vi "plot_usr_seq.vi"(1 "User-defined sequence":string[][](table)) -> (0 "Sequence Preview":cluster{dbl[], dbl[]}[](graph))   [LabVIEW 2014]
panel:
  in  "Boolean":bool=TRUE
  out "Total sequence time (sec)":dbl
  out "vapor flow":dbl
  out "gas flow":dbl
  out "Pressure":dbl
  out "light up\ncurrent step":bool[](array[boolean])
  in  "Run sequence":bool
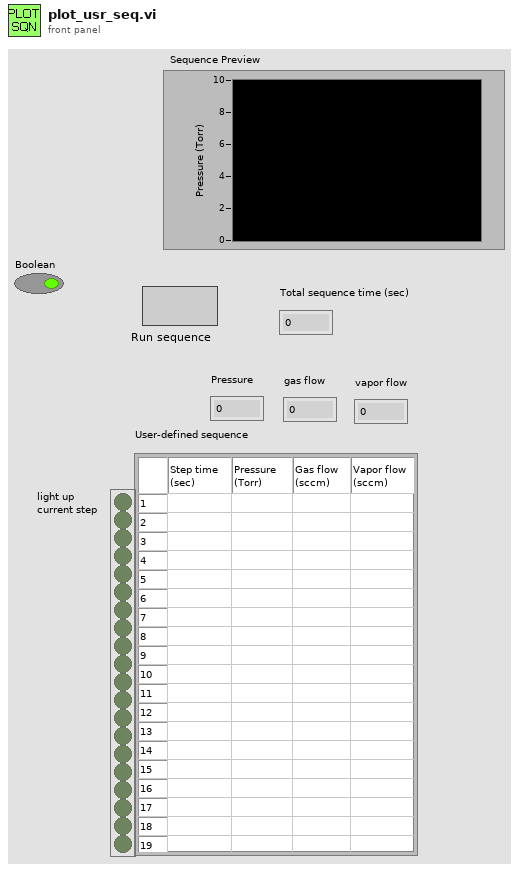
[diagram p1: front panel]
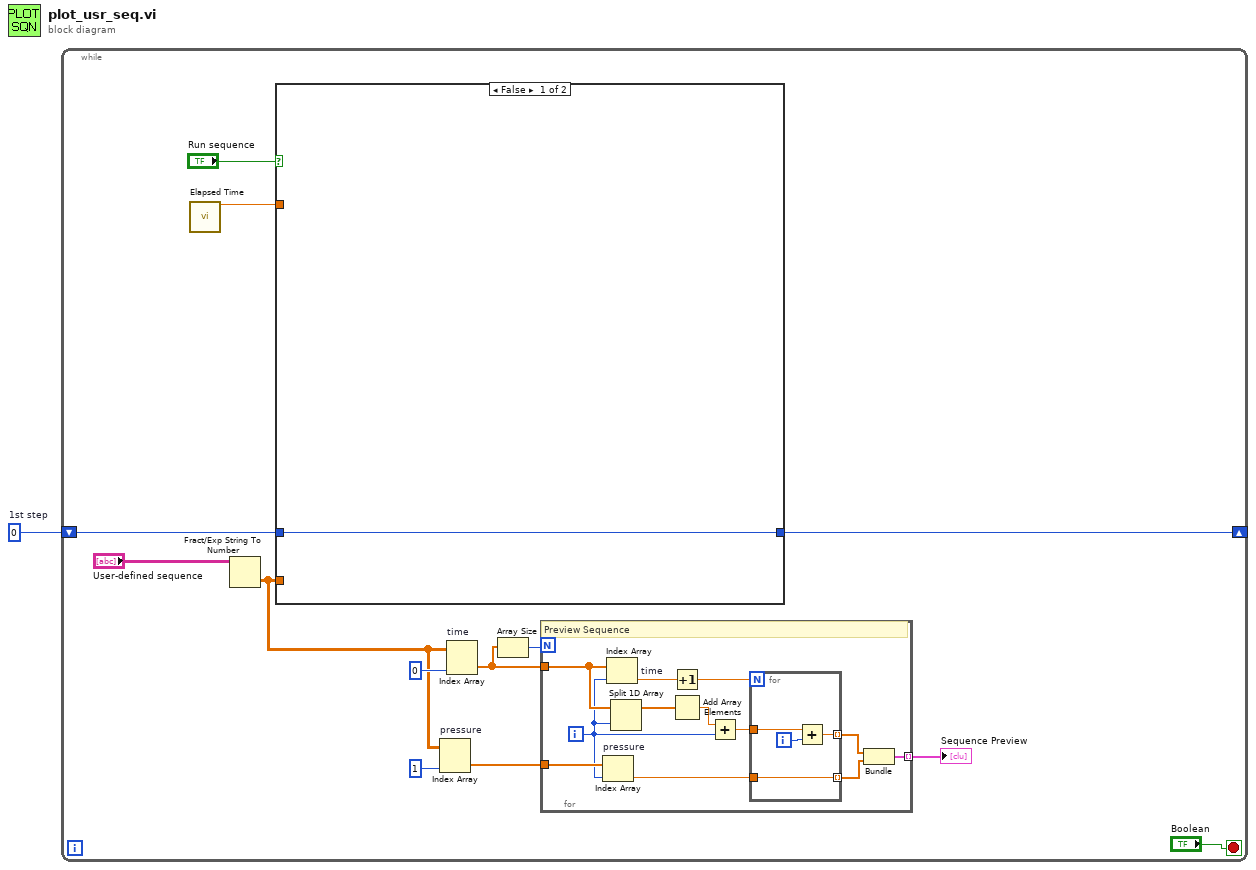
[diagram p0: block diagram]
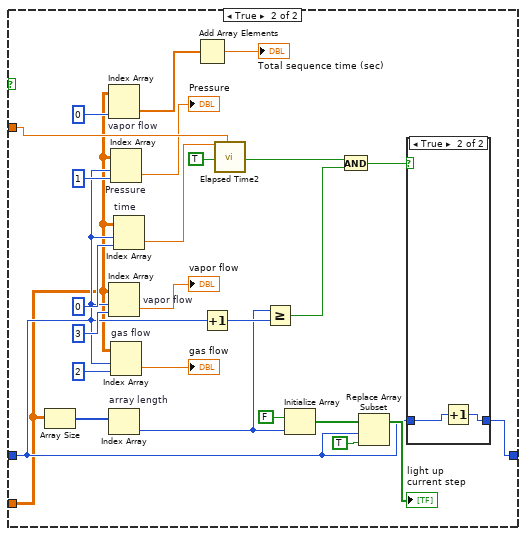
[diagram p2: hidden frame]
diagram:
  w1 = 0  # 1st step
  n1 = while {
    shift-right: [w13] -> _
    shift-left: w1 -> [w12]
    stop <- "Boolean" stop-if-true
    n2 = call "Elapsed Time"() -> ("Present (s)"=w14:dbl)  [unwired: 12 in, 7 out]
    n3 = Fract/Exp String To Number(string="User-defined sequence") -> (number=w6:dbl[][])  [unwired: 3 in, 1 out]
    n4 = case shown="False" "Run sequence" {
      tunnel: w14 -> [_ w35]
      tunnel: [w31 w50] -> w13
      tunnel: w12 -> [w31 w39]
      tunnel: w6 -> [_ w32]
      frame False {
      }
      frame True {
        n5 = Array Size(array=w32) -> (size(s)=w57:i32[])
        n6 = Index Array "vapor flow"(array=w32, index (col)=0 ("disabled index (col)")) -> (element=w37:dbl[])  [unwired: 1 in]
        n7 = Index Array "vapor flow"(array=w32, index (row)=w39, index (col)=3 ("disabled index (col)")) -> (element=→"vapor flow":dbl)
        n8 = Index Array "array length"(array=w57) -> (element=w47:i32)  [unwired: 1 in]
        n9 = Index Array "Pressure"(array=w32, index (row)=w39, index (col)=1 ("disabled index (col)")) -> (element=→"Pressure":dbl)
        n10 = Index Array "gas flow"(array=w32, index (row)=w39, index (col)=2 ("disabled index (col)")) -> (element=→"gas flow":dbl)
        n11 = Index Array "time"(array=w32, index (row)=w39, index (col)=0) -> (element=w55:dbl)
        n12 = Add Array Elements(numeric array=w37) -> (sum=→"Total sequence time (sec)":dbl)
        n13 = Increment(x=w39) -> (x+1=w48:i32)
        n14 = call "Elapsed Time2"("Time Target (s)"=w55, "Auto Reset"=TRUE, "Set Start Time (s)"=w35) -> ("Time has Elapsed"=w44:bool)  [unwired: 9 in, 7 out]
        n15 = Greater Or Equal?(x=w47, y=w48) -> (x >= y?=w46:bool)
        n16 = Initialize Array(FALSE ("new element/subarray"), w47) -> (w54:bool[])
        n17 = And(x=w44, y=w46) -> (x .and. y?=w45:bool)
        n18 = Replace Array Subset(array=w54, new element=TRUE ("new element/subarray"), index=w39) -> (→"light up\ncurrent step":bool[])
        n19 = case shown="True" w45 {
          tunnel: [w58 w59] -> w50
          tunnel: w39 -> [w58 w60]
          frame False {
          }
          frame True {
            n20 = Increment(x=w60) -> (x+1=w59:i32)
          }
        }
      }
    }
    n21 = Index Array "pressure"(array=w6, index (col)=1 ("disabled index (col)")) -> (element=w5:dbl[])  [unwired: 1 in]
    n22 = Index Array "time"(array=w6, index (col)=0 ("disabled index (col)")) -> (element=w3:dbl[])  [unwired: 1 in]
    n23 = Array Size(array=w3) -> (size(s)=w2:i32)
    n24 = for {
      N: w2 -> [_]
      tunnel: w3 -> [w22]
      tunnel: w5 -> [w26]
      tunnel: [w24] -> w4 mode=indexing
      i -> [w19]
      # "Preview Sequence"
      n25 = Index Array "pressure"(array=w26, index=w19) -> (element=w25:dbl)
      n26 = Index Array "time"(array=w22, index=w19) -> (element=w18:dbl)
      n27 = Split 1D Array(array=w22, index=w19) -> (first subarray=w21:dbl[])  [unwired: 1 out]
      n28 = Increment(x=w18) -> (x+1=w17:dbl)
      n29 = Add Array Elements(numeric array=w21) -> (sum=w20:dbl)
      n30 = Add(x=w20, y=w19) -> (x+y=w23:dbl)
      n31 = for {
        N: w17 -> [_]
        tunnel: [w30] -> w15 mode=indexing
        tunnel: w25 -> [w30]
        tunnel: [w27] -> w16 mode=indexing
        tunnel: w23 -> [w29]
        i -> [w28]
        n32 = Add(x=w29, y=w28) -> (x+y=w27:dbl)
      }
      n33 = Bundle(w16, w15) -> (w24:cluster{dbl[], dbl[]})  [unwired: 1 in]
    }
    "Sequence Preview" <- w4
  }
